vi "fgv_laser shutter ops.vi"(7 "FGV Actions":T1, 8 "error in (no error)":errorcluster, 10 "Shutter state":bool, 11 "Operate Shutter":bool) -> (0 "error out":errorcluster, 2 "Shutter state [OUT]":bool, 3 "Operate Shutter [OUT}":bool)   [LabVIEW 2020]
uses:
  Typedefs/fgv_actions.ctl
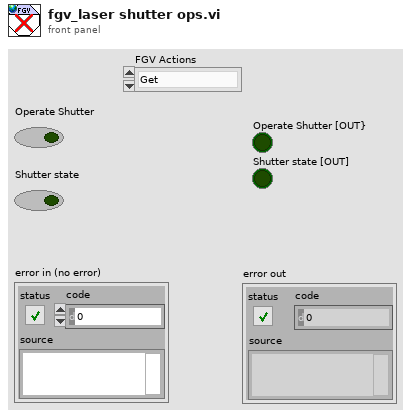
[diagram p1: front panel]
types:
  T1 = typedef "fgv_actions.ctl" = enum16{"Get", "Set"}
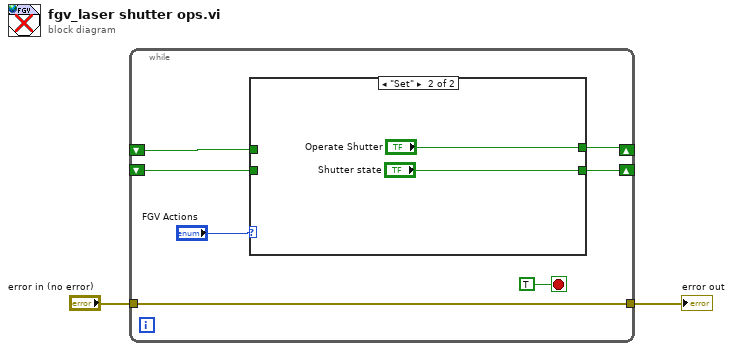
[diagram p0: block diagram]
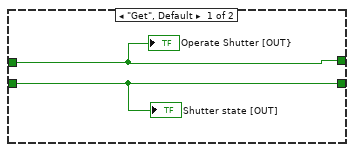
[diagram p2: hidden frame]
diagram:
  n1 = while {
    shift-right: [w7] -> _
    shift-left: _ -> [w6]
    shift-right: [w5] -> _
    shift-left: _ -> [w4]
    tunnel: "error in (no error)" -> [w3]
    tunnel: [w3] -> w1
    stop <- TRUE stop-if-true
    n2 = case shown="\"Set\"" "FGV Actions" {
      tunnel: [w11 "Operate Shutter"] -> w7
      tunnel: w6 -> [w11 _]
      tunnel: [w10 "Shutter state"] -> w5
      tunnel: w4 -> [w10 _]
      frame "Get", Default {
        "Operate Shutter [OUT}" <- w11
        "Shutter state [OUT]" <- w10
      }
      frame "Set" {
      }
    }
  }
  "error out" <- w1
